vi "WPI_RelaySafetyError.vi"(0 "RelayDevRef":T1={"DevStatus"={"status"=FALSE, "code"=0, "source"=""}, "Relay Channel"=enum."Relay 2", "Relay Direction"=enum."Both directions"}) -> (4 "RelayDevRef 2":T1={"DevStatus"={"status"=FALSE, "code"=0, "source"=""}, "Relay Channel"=enum."Relay 2", "Relay Direction"=enum."Both directions"})   [LabVIEW 2017]
doc: "This subVI does two things:\n1. It builds up output specific information to help locate the problem.\n2. It calls the FRC Build Error, so all the information gets passed to the Driver Station."
uses:
  <vilib>/Rock Robotics/WPI/Relay/WPI_RelayDevRef.ctl
  <vilib>/Rock Robotics/SystemInterfaces/DIO/FPGA_DIORelayChannel.ctl
  <vilib>/Rock Robotics/WPI/Relay/WPI_RelayDirection.ctl
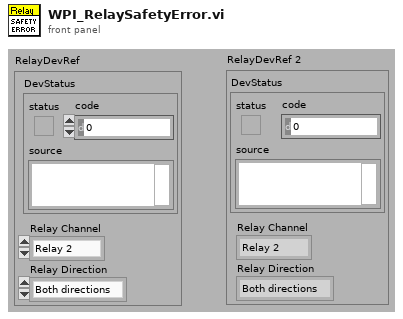
[diagram p1: front panel]
types:
  T1 = typedef "WPI_RelayDevRef.ctl" = cluster{"DevStatus":errorcluster, "Relay Channel":T2, "Relay Direction":T3}
  T2 = typedef "FPGA_DIORelayChannel.ctl" = enum8{"Relay 0", "Relay 1", "Relay 2", "Relay 3", "Invalid"}
  T3 = typedef "WPI_RelayDirection.ctl" = enum16{"Both directions", "Forward only", "Reverse only"}
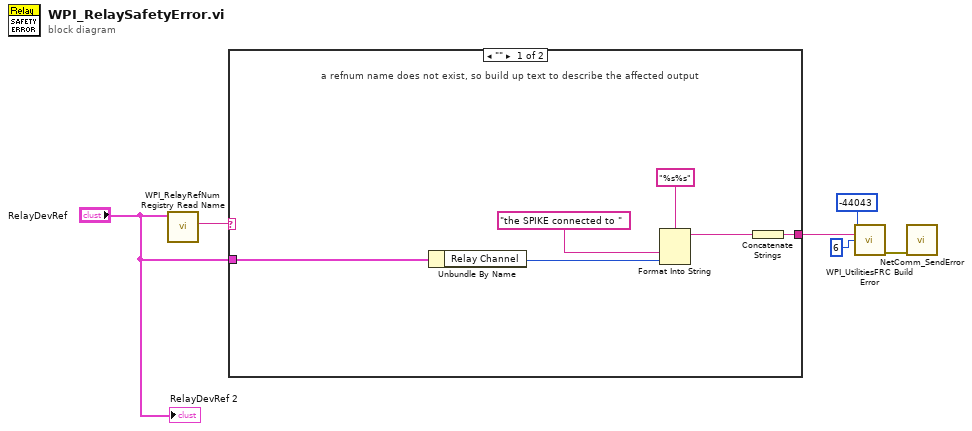
[diagram p0: block diagram]
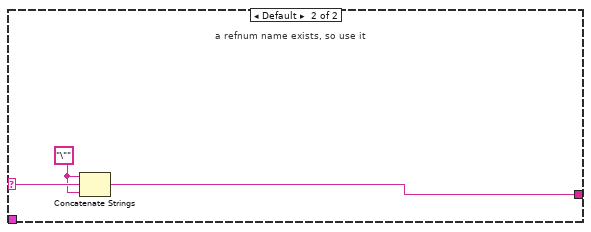
[diagram p2: hidden frame]
diagram:
  n1 = call <vilib>:"WPI_RelayRefNum Registry Read Name.vi"("RelayDevRef"="RelayDevRef") -> ("refnum name"=w4:string)  [unwired: 1 in, 9 out]
  n2 = case shown="\"\"" w4 {
    selector: w4 -> [_ w15]
    tunnel: [w11 w14] -> w3
    tunnel: "RelayDevRef" -> [w10 _]
    frame "" {
      # "a refnum name does not exist, so build up text to describe the affected output"
      n3 = Unbundle By Name(w10) -> ("Relay Channel"=w7:T2)
      n4 = Format Into String(format string="%s%s", "the SPIKE connected to " ("format string"), w7) -> (resulting string=w12:string)  [unwired: 2 in, 1 out]
      n5 = Concatenate Strings(w12) -> (w11:string)
    }
    frame Default {
      w13 = "\"" ("string")
      # "a refnum name exists, so use it"
      n6 = Concatenate Strings(w13, w15, w13) -> (w14:string)
    }
  }
  n7 = call <vilib>:"WPI_UtilitiesFRC Build Error.vi"("error code"=-44043 ("code"), "extra error text"=w3, "chain levels to remove (1)"=6) -> ("error out"=w1:errorcluster)  [unwired: 3 in, 9 out]
  n8 = call <vilib>:"NetComm_SendError.vi"("error in (no error)"=w1) -> ()  [unwired: 11 in]
  "RelayDevRef 2" <- "RelayDevRef"
